vi "Read MultiPointParams.vi"(8 "error in (no error)":errorcluster, 11 "NISTSamplerPluginsBase in":refnum<class "SamplerPluginsBase.lvclass">) -> (0 "error out":errorcluster, 2 "MultiPointParams":T1, 3 "NISTSamplerPluginsBase out":refnum<class "SamplerPluginsBase.lvclass">)   [LabVIEW 2014, in "SamplerPlugins.lvlib" / "SamplerPluginsBase.lvclass"]
uses:
  SamplerPluginsBase.lvclass
  TypeDefs/MultiPointParams.ctl
  SamplerPluginsBase.lvclass/SamplerPluginsBase.ctl
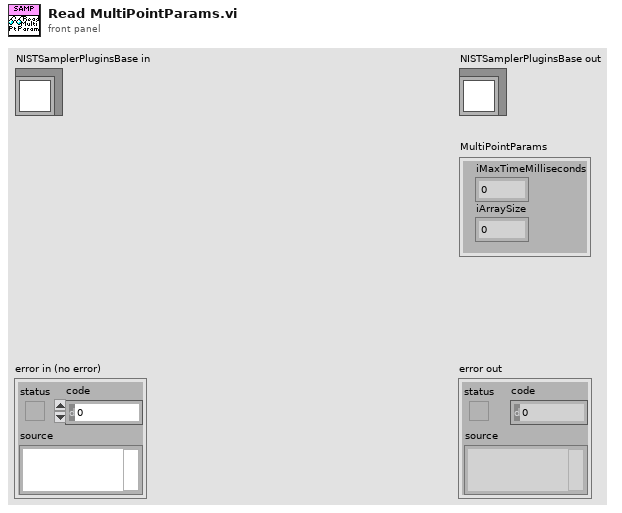
[diagram p1: front panel]
types:
  T1 = typedef "SamplerPlugins.lvlib/SamplerPluginsBase.lvclass/MultiPointParams.ctl" = cluster{"iMaxTimeMilliseconds":i32, "iArraySize":i32}
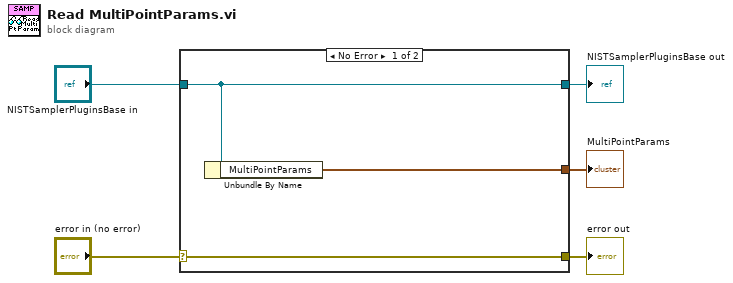
[diagram p0: block diagram]
diagram:
  n1 = case shown="No Error" "error in (no error)" {
    selector: "error in (no error)" -> [w8 w9]
    tunnel: [w8 w9] -> w4
    tunnel: [w7 w10] -> w2
    tunnel: "NISTSamplerPluginsBase in" -> [w7 w10]
    tunnel: [w6 _] -> w1
    frame No Error {
      n2 = Unbundle By Name(w7) -> ("MultiPointParams"=w6:T1)
    }
    frame Error {
    }
  }
  "error out" <- w4
  "NISTSamplerPluginsBase out" <- w2
  "MultiPointParams" <- w1
